vi "gen_digital_blank.vi"(7 "sampling rate":dbl format="%#_6p", 8 "waveform length":i32, 11 "On / Off":bool) -> (3 "digital waveform":digitalwaveform(waveform)={"t0"=timestamp(0 s since 1904-01-01), "dt"=0.0, "Y"={"transitions"=[], "data"=[]}, "error"={"status"=FALSE, "code"=37421928, "source"=""}})   [LabVIEW 2019]
uses:
  <vilib>/Waveform/DWDTOps.llb/DWDT Analog to Digital.vi
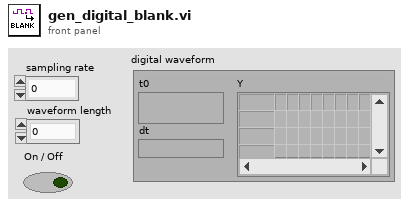
[diagram p1: front panel]
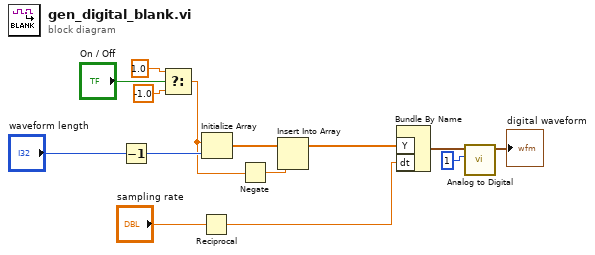
[diagram p0: block diagram]
diagram:
  n1 = Decrement(x="waveform length") -> (x-1=w5:i32)
  n2 = Select(t=1.0, s="On / Off", f=-1.0) -> (s? t:f=w2:dbl)
  n3 = Reciprocal(x="sampling rate") -> (1/x=w10:dbl)
  n4 = Initialize Array(w2, w5) -> (w4:dbl[])
  n5 = Negate(x=w2) -> (-x=w3:dbl)
  n6 = Insert Into Array(array=w4, new element=w3) -> (w1:dbl[])  [unwired: 1 in]
  n7 = Bundle By Name("Y"=w1, "dt"=w10) -> (w11:waveform(dbl))  [unwired: 1 in]
  n8 = call-poly <vilib>:"Analog to Digital.vi"("resolution (16 bit)"=1, "analog waveform"=w11) -> ("digital waveform"=→"digital waveform":digitalwaveform)  [unwired: 6 in, 3 out]
